vi "Proceed Dialog.vi"(8 "PID In Range?":bool) -> (0 "Wait To Settle":bool, 1 "Force Nexzt Step":bool, 2 "Stay On Current Step":bool)   [LabVIEW 2018]
panel:
  in  "Force Nexzt Step":bool
  in  "Stay On Current Step":bool
  # "Test fell out of tolerance..."
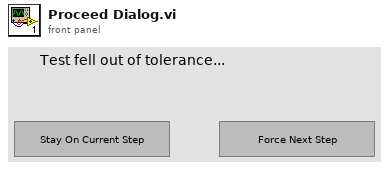
[diagram p1: front panel]
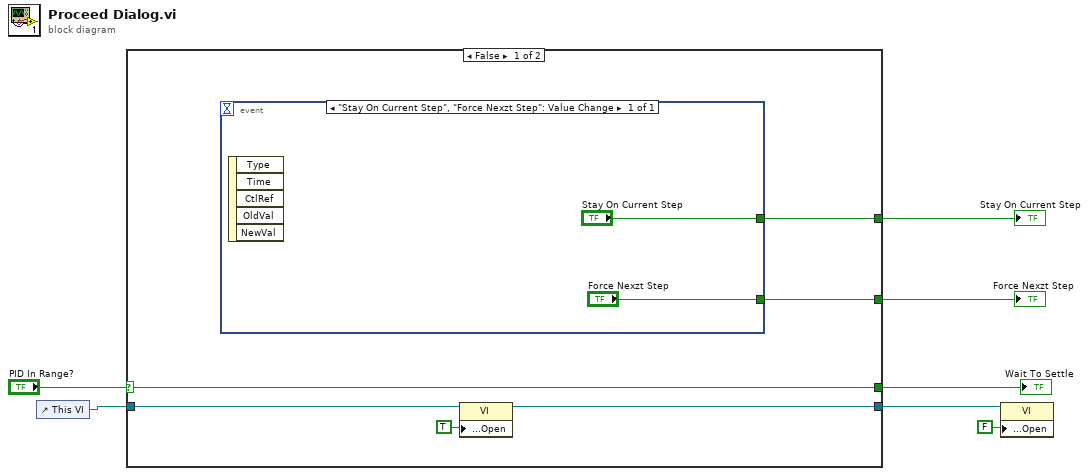
[diagram p0: block diagram]
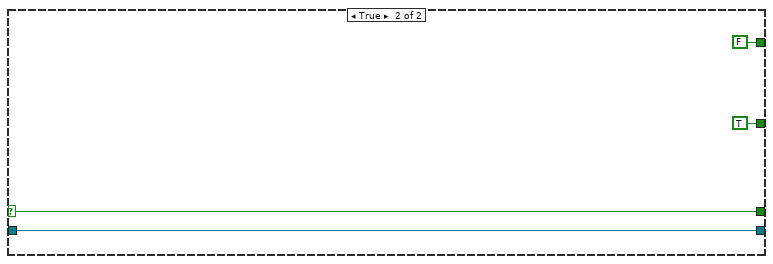
[diagram p2: hidden frame]
diagram:
  n1 = control-ref of="This VI"() -> (w2:refnum<vi>)
  n2 = case shown="False" "PID In Range?" {
    selector: "PID In Range?" -> [w11 w19]
    tunnel: [w13 FALSE ("Stay On Current Step")] -> w7
    tunnel: [w12 TRUE ("Force Nexzt Step")] -> w6
    tunnel: [w11 w19] -> w4
    tunnel: [w10 w16] -> w3
    tunnel: w2 -> [w9 w16]
    frame False {
      n3 = event shown="[0] \"Stay On Current Step\", \"Force Nexzt Step\": Value Change" {
        selector: _ -> [_]
        dyn-events: _ -> [_]
        timeout: _ -> [_]
        tunnel: ["Stay On Current Step"] -> w13
        tunnel: ["Force Nexzt Step"] -> w12
        event "Stay On Current Step", "Force Nexzt Step": Value Change {
          n4 = event-data() -> ()  [unwired: 1 in, 5 out]
        }
      }
      n5 = property class="VI"(reference=w9, "Front Panel.Open"=TRUE ("Front Panel Window:Open")) -> (reference out=w10:refnum<vi>)  [unwired: 1 in, 1 out]
    }
    frame True {
    }
  }
  "Stay On Current Step" <- w7
  "Force Nexzt Step" <- w6
  "Wait To Settle" <- w4
  n6 = property class="VI"(reference=w3, "Front Panel.Open"=FALSE ("Front Panel Window:Open")) -> ()  [unwired: 1 in, 2 out]
